vi "Cleanup.vi"(8 "error in (no error)":errorcluster, 11 "SQLite in":refnum<class "SQLite.lvclass">) -> (0 "error out":errorcluster)   [LabVIEW 2022 SP3, in "Conditum SQLite.lvlib" / "SQLite.lvclass"]
uses:
  SQLite.lvclass
  SQLite.lvclass/SQLite.ctl
  <vilib>/drjdpowell/SQLite Library/SQL Connection/Connection.lvclass
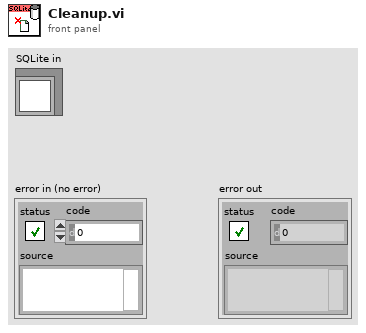
[diagram p1: front panel]
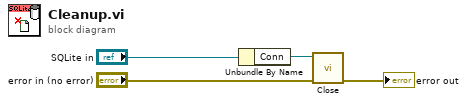
[diagram p0: block diagram]
diagram:
  n1 = Unbundle By Name("SQLite in") -> ("Conn"=w3:refnum<class "Connection.lvclass">)
  n2 = call-dynamic "Close.vi"("error in (no error)"="error in (no error)", "SQLite Connection in"=w3) -> ("error out"=→"error out":errorcluster)  [unwired: 9 in]
